vi "MathScript Waveform Simulator.vi"() -> ()   [LabVIEW 2017]
uses:
  <vilib>/imath/engines/lvmath2/RunTimeEngine/Managers/WorkSpace/UID Generator.vi
  <vilib>/imath/engines/lvmath2/RunTimeEngine/RangeToken/NIMS_Range.vi
  <instcachedir>/0/NIMS_Range_69CB9AAD882742A19CF7E739BE79952C.lvgen/NIMS_Range_69CB9AAD882742A19CF7E739BE79952C_000.vi
  <vilib>/imathl/engines/lvmath/Functions/Error Handling/Create Error.vi
  <vilib>/imath/engines/lvmath2/RunTimeEngine/RunTimeType/NIMS_RunTimeType_From StrictType (excl LVString).vi
  <instcachedir>/0/NIMS_RunTimeType_From StrictType (excl LVString)_1019F277F0A747EDBCA0F6C52CA54500.lvgen/NIMS_RunTimeType_From StrictType (excl LVString)_1019F277F0A747EDBCA0F6C52CA54500_000.vi
  <vilib>/imath/engines/lvmath2/RunTimeEngine/LocalVariableDefStatement/MC_LocalVariableDefStatement_Display.vi
  <vilib>/imath/engines/lvmath2/RunTimeEngine/Managers/SymbolTable/Clear UID.vi
  <vilib>/imath/engines/lvmath2/RunTimeEngine/NodeEndStatement/NIMS_NodeEndStatement_Output.vi
  <instcachedir>/0/NIMS_NodeEndStatement_Output_53EC0D466D134D7ABD903AC30B43404B.lvgen/NIMS_NodeEndStatement_Output_53EC0D466D134D7ABD903AC30B43404B_005.vi
  <vilib>/imath/engines/lvmath2/RunTimeEngine/ErrorHandling/NIMS_Finalize Error.vi
  <vilib>/imath/engines/lvmath2/RunTimeEngine/Managers/SymbolTable/NIMS_WorkSpace.lvlib
panel:
  out "Displacement":dbl[](array[numeric])
  out "Time":dbl[](array[numeric])
  in  "Amplitude":dbl
  in  "Frequency":dbl
  in  "Sampling Frequency":dbl
  in  "Number of Samples":dbl
  out "XY Graph":cluster{"t":dbl[], "x":dbl[]}(graph)
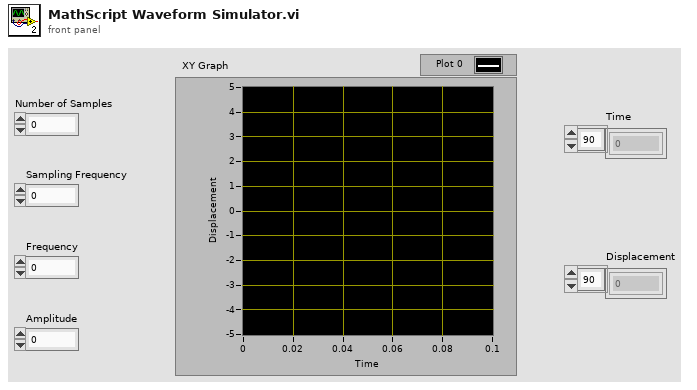
[diagram p1: front panel]
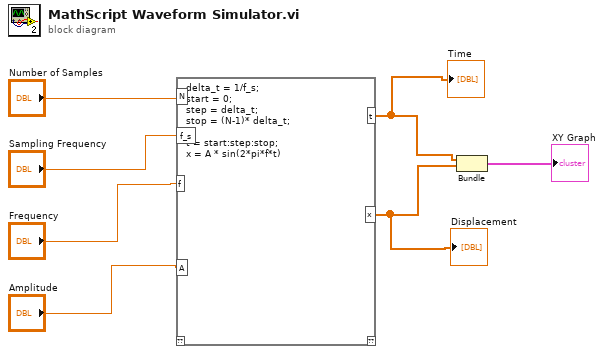
[diagram p0: block diagram]
diagram:
  n1 = mathscript code="delta_t = 1/f_s;\nstart = 0;\nstep = delta_t;\nstop = (N-1)* delta_t;\n\nt = start:step:stop; \nx = A * sin(2*pi*f*t)"("N"="Number of Samples", "f_s"="Sampling Frequency", "f"="Frequency", "A"="Amplitude") -> ("t"=w2:dbl[], "x"=w1:dbl[])  [unwired: 1 in, 1 out]
  "Time" <- w2
  "Displacement" <- w1
  n2 = Bundle("t"=w2, "x"=w1) -> (→"XY Graph":cluster{"t":dbl[], "x":dbl[]})  [unwired: 1 in]
